vi "test_Read Bool Register Value.vi"(8 "error in (no error)":errorcluster, 11 "TestCase in":refnum<class "FPGA Register IO Tests.lvclass">) -> (0 "error out":errorcluster, 3 "TestCase out":refnum<class "FPGA Register IO Tests.lvclass">)   [LabVIEW 2021, in "FPGA Register IO Tests.lvclass"]
uses:
  FPGA Register IO Tests.lvclass
  FPGA Register IO Tests.lvclass/FPGA Register IO Tests.ctl
  APIs/FPGA Register IO/Read Methods/Read Data Register/Instances/Read Boolean.vi
  APIs/FPGA Register IO/Utilities/Find Register Offset.vi
  APIs/FPGA Register IO/SubVIs/Check Register Data Store.vi
  APIs/FPGA Register IO/Error Handling/Error 6001.vi
  APIs/FPGA Register IO/Error Handling/Error 6000.vi
  APIs/FPGA Register IO/Error Handling/Error 6002.vi
  APIs/FPGA Register IO/Error Handling/Error 6003.vi
  <vilib>/FPGAPlugInAG/Dynamic/niLvFpga_Close_Dynamic.vi
  <vilib>/rvi/interface/nirviCloseFPGA/nirviCloseFPGA.xnode
  <vilib>/addons/_JKI Toolkits/VI Tester/TestCase.llb/TestCase.lvclass
  APIs/FPGA Register IO/FPGA Register IO.lvlib
  C:/Program Files/National Instruments/LabVIEW 2021/vi.lib/addons/_JKI Toolkits/VI Tester/TestCase.llb/TestCase.lvclass
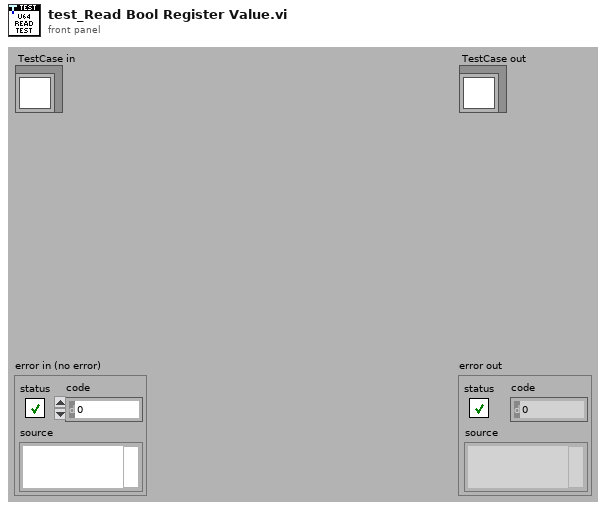
[diagram p1: front panel]
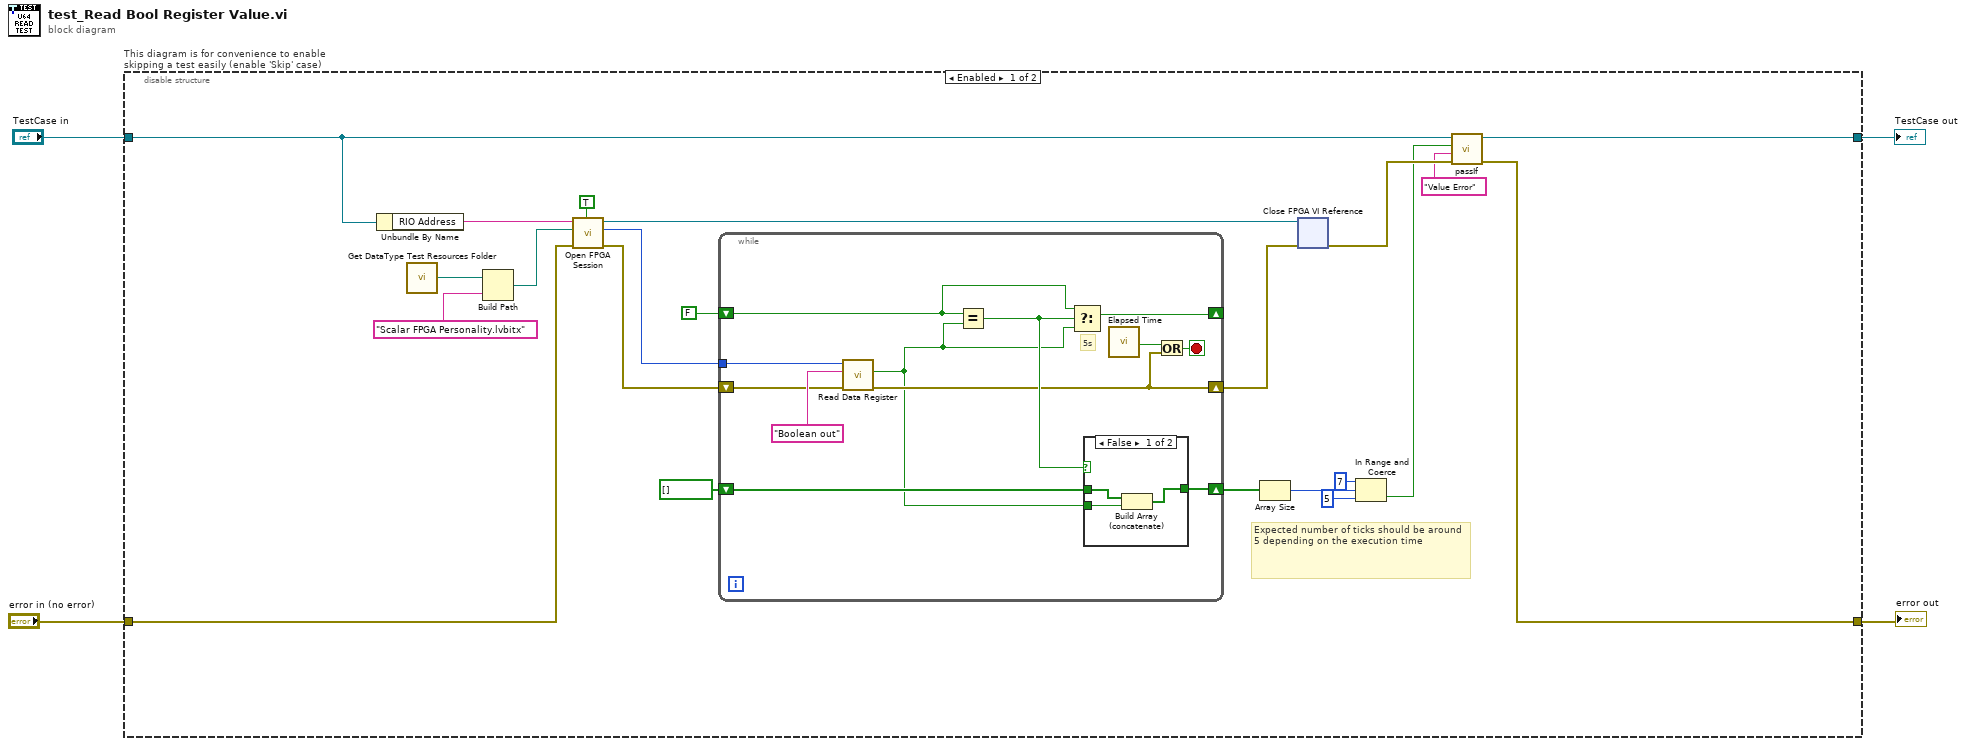
[diagram p0: block diagram]
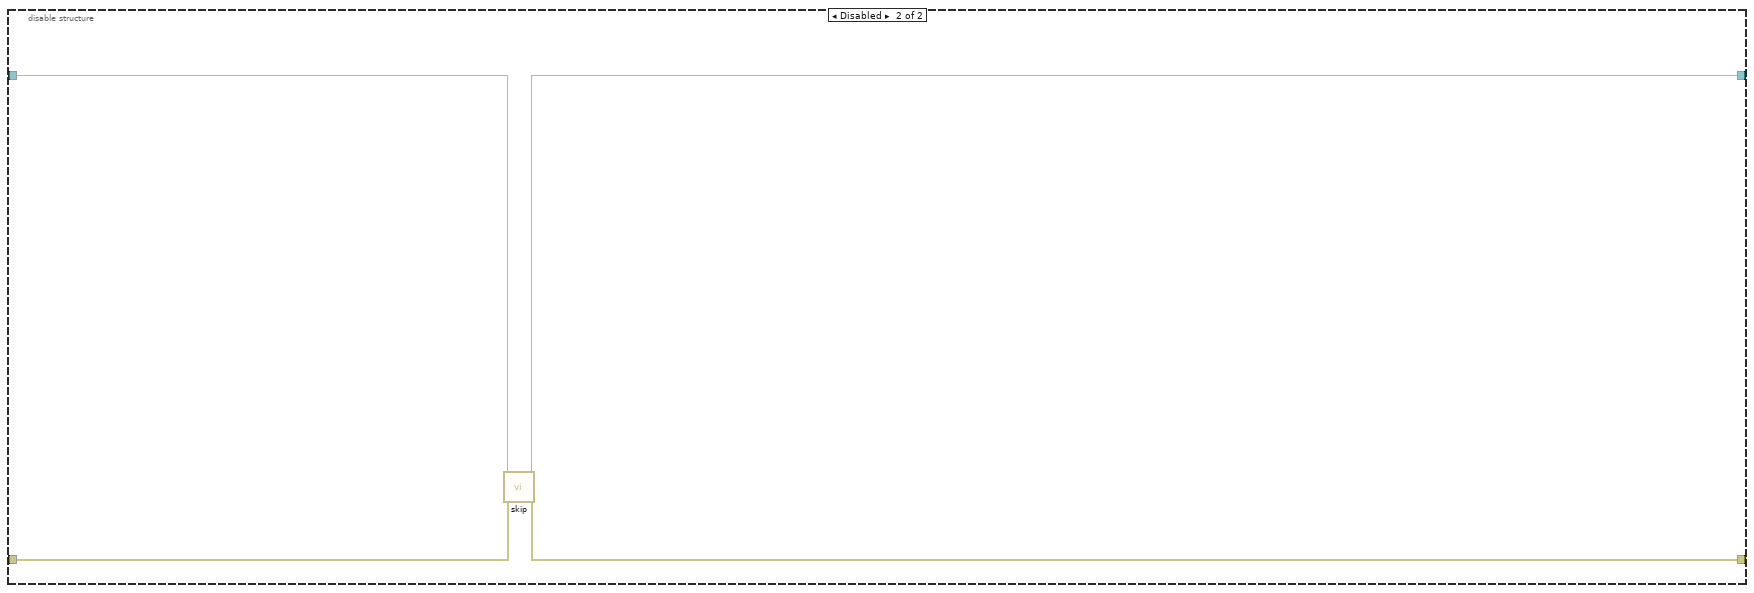
[diagram p3: hidden frame]
diagram:
  n1 = disable-structure "This diagram is for convenience to enable skipping a test easily (enable 'Skip' case)" shown="Enabled" {
    disable-tunnel: "TestCase in" -> [w16 w46]
    disable-tunnel: [w11 w44] -> w1
    disable-tunnel: [w10 w45] -> w3
    disable-tunnel: "error in (no error)" -> [w17 w43]
    frame Enabled {
      # "Expected number of ticks should be around 5 depending on the execution time"
      n2 = Unbundle By Name(w16) -> ("RIO Address"=w19:string)
      n3 = call "Get DataType Test Resources Folder.vi"() -> ("path"=w14:path)
      n4 = Build Path(base path=w14, name or relative path="Scalar FPGA Personality.lvbitx") -> (appended path=w18:path)
      n5 = call "Open FPGA Session.vi"("run when loaded (T)"=TRUE ("Run When Loaded (T)"), "error in"=w17, "bitfile path"=w18, "device address"=w19) -> ("error out"=w24:errorcluster, "session out"=w23:u32, "bitfile reference out"=w22:refnum<k20>)  [unwired: 5 in]
      n6 = while {
        tunnel: w23 -> [w33]
        shift-right: [w28] -> w21
        shift-left: w24 -> [w31]
        shift-right: [w37] -> _
        shift-left: FALSE ("value out") -> [w38]
        shift-right: [w35] -> w25
        shift-left: bool[] [] -> [w34]
        stop <- w30 stop-if-true
        # "5s"
        n7 = call-poly "Read Data Register.vi"("error in"=w31, "register name"="Boolean out" ("registerName"), "session in"=w33) -> ("error out"=w28:errorcluster, "value out"=w27:bool)  [unwired: 6 in, 1 out]
        n8 = Equal?(x=w38, y=w27) -> (x = y?=w36:bool)
        n9 = Select(t=w38, s=w36, f=w27) -> (s? t:f=w37:bool)
        n10 = case shown="False" w36 {
          tunnel: w27 -> [w41 _]
          tunnel: [w40 w42] -> w35
          tunnel: w34 -> [w39 w42]
          frame False {
            n11 = Build Array (concatenate)(w39, w41) -> (w40:bool[])
          }
          frame True {
          }
        }
        n12 = call "Elapsed Time"() -> ("Time has Elapsed"=w29:bool)  [unwired: 12 in, 7 out]
        n13 = Or(x=w29, y=w28) -> (x .or. y?=w30:bool)
      }
      n14 = Array Size(array=w25) -> (size(s)=w8:i32)
      n15 = xnode "Close FPGA VI Reference"("FPGA VI Reference In"=w22, "error in"=w21) -> ("error out"=w15:errorcluster)
      n16 = In Range and Coerce(upper limit=7, x=w8, lower limit=5) -> (In Range?=w5:bool)  [unwired: 1 out]
      n17 = call-dynamic "passIf.vi"("error in (no error)"=w15, "message (\"\")"="Value Error" ("message (\"\")"), "pass"=w5, "TestCase in"=w16) -> ("error out"=w10:errorcluster, "TestCase out"=w11:refnum<class "FPGA Register IO Tests.lvclass">)  [unwired: 6 in]
    }
    frame Disabled {
      # "skip test result while test is under development"
      n18 = call <vilib>:"skip.vi"("error in (no error)"=w43, "TestCase in"=w46) -> ("error out"=w45:errorcluster, "TestCase out"=w44:refnum<class "FPGA Register IO Tests.lvclass">)  [unwired: 8 in]
    }
  }
  "error out" <- w3
  "TestCase out" <- w1
